vi "Q8381 MEASURE.vi"(1 "Meas mode":u16(ring) items=["STOP", "SINGLE", "REPEAT"], 2 "GPIB Address":u16=8 max=31 step=1, 3 "VISA resource name":refnum<visa-resource-name>) -> (0 "GPIB Status":bool)   [LabVIEW 2017]
doc: "Meas mode: \n 0: stop, 1: single, 2: repeat."
panel:
  out "Program Code":string
  # "MEASURE mode"
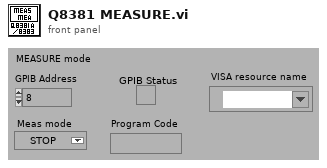
[diagram p1: front panel]
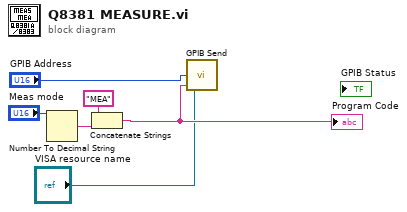
[diagram p0: block diagram]
diagram:
  n1 = Number To Decimal String(number="Meas mode") -> (decimal integer string=w5:string)  [unwired: 1 in]
  n2 = Concatenate Strings("MEA", w5) -> (w3:string)
  "Program Code" <- w3
  n3 = call "GPIB Send.vi"("Command String"=w3, "Address"="GPIB Address", "VISA resource name"="VISA resource name") -> ()  [unwired: 1 out]
